vi "Animation Demo.vi"() -> ()   [LabVIEW 2017]
panel:
  in  "Delay":u32=100
  in  "Menu Button":bool
  in  "Menu":enum32{"Page 1", "Page 2"}(tab)
  out "Hardware Config Button":bool
  out "Setup Button":bool
  out "Home Button":bool
  in  "Main Display":enum32{"Page 1", "Page 2"}(tab)
  out "Main Data Display":dbl[](graph)
  in  "stop":bool
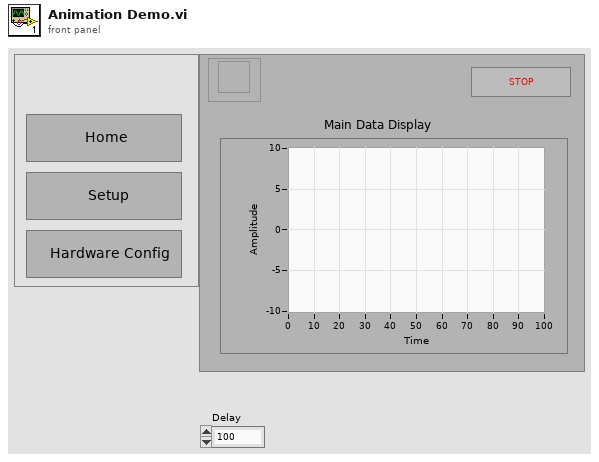
[diagram p1: front panel]
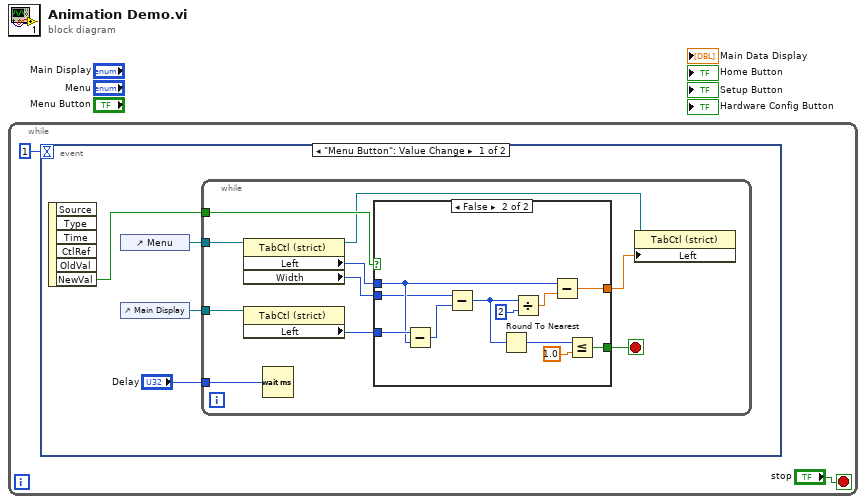
[diagram p0: block diagram]
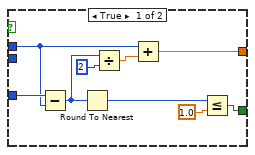
[diagram p2: hidden frame]
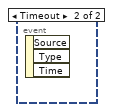
[diagram p3: hidden frame]
diagram:
  n1 = while {
    stop <- "stop" stop-if-true
    n2 = event shown="[0] \"Menu Button\": Value Change" {
      selector: _ -> [_ _]
      dyn-events: _ -> [_ _]
      timeout: 1 -> [_ _]
      event "Menu Button": Value Change {
        n3 = event-data() -> ("NewVal"=w4:bool)  [unwired: 1 in, 5 out]
        n4 = control-ref of="Menu"() -> (w6:refnum<vi>)
        n5 = control-ref of="Main Display"() -> (w5:refnum<vi>)
        n6 = while {
          tunnel: w4 -> [w15]
          tunnel: w6 -> [w10]
          tunnel: w5 -> [w9]
          tunnel: "Delay" -> [w7]
          stop <- w11 stop-if-true
          n7 = property on="Property Node" class="TabCtl (strict)"(reference=w10) -> (reference out=w8:refnum<vi>, "Left"=w13:i32, "Width"=w16:u32)  [unwired: 1 in, 1 out]
          n8 = property on="Property Node" class="TabCtl (strict)"(reference=w9) -> ("Left"=w14:i32)  [unwired: 1 in, 2 out]
          n9 = Wait (ms)(milliseconds to wait=w7) -> ()  [unwired: 1 out]
          n10 = case shown="False" w15 {
            tunnel: w16 -> [_ w28]
            tunnel: w14 -> [w23 w34]
            tunnel: w13 -> [w17 w29]
            tunnel: [w22 w33] -> w12
            tunnel: [w18 w30] -> w11
            frame True {
              n11 = Subtract(x=w23, y=w17) -> (x-y=w19:i32)
              n12 = Round To Nearest(number=w19) -> (nearest integer value=w20:i32)
              n13 = Divide(x=w19, y=2) -> (x/y=w25:dbl)
              n14 = Add(x=w17, y=w25) -> (x+y=w22:dbl)
              n15 = Less Or Equal?(x=w20, y=1.0) -> (x <= y?=w18:bool)
            }
            frame False {
              n16 = Subtract(x=w34, y=w29) -> (x-y=w27:i32)
              n17 = Subtract(x=w28, y=w27) -> (x-y=w26:u32)
              n18 = Round To Nearest(number=w26) -> (nearest integer value=w31:u32)
              n19 = Divide(x=w26, y=2) -> (x/y=w36:dbl)
              n20 = Subtract(x=w29, y=w36) -> (x-y=w33:dbl)
              n21 = Less Or Equal?(x=w31, y=1.0) -> (x <= y?=w30:bool)
            }
          }
          n22 = property on="Property Node" class="TabCtl (strict)"(reference=w8, "Left"=w12) -> ()  [unwired: 1 in, 2 out]
        }
      }
      event Timeout {
        n23 = event-data() -> ()  [unwired: 1 in, 3 out]
      }
    }
  }
